vi "HandleTCPError.vi"(8 "error in (no error)":errorcluster, 10 "NoErrorMessage":refnum<class "Message.lvclass">, 11 "ServiceManager-Comms in":refnum<class "ServiceManager-Comms.lvclass">) -> (0 "error out":errorcluster, 3 "ServiceManager-Comms out":refnum<class "ServiceManager-Comms.lvclass">)   [LabVIEW 2020, in "ServiceManager-Comms.lvlib" / "ServiceManager-Comms.lvclass"]
uses:
  ServiceManager-Comms.lvclass
  C:/Program Files (x86)/National Instruments/LabVIEW 2020/vi.lib/ActorFramework/Actor/Actor.lvclass
  <vilib>/ActorFramework/Message/Message.lvclass
  ServiceManager-Comms Messages/WaitForConnect Msg/WaitForConnect Msg.lvclass
  C:/Program Files (x86)/National Instruments/LabVIEW 2020/vi.lib/ActorFramework/Message/Message.lvclass
  <vilib>/ActorFramework/Actor/Actor.lvclass/Actor.ctl
  <vilib>/ActorFramework/Message Enqueuer/Message Enqueuer.lvclass/Message Enqueuer.ctl
  <vilib>/ActorFramework/Message Enqueuer/Init from Existing Queue.vi
  <vilib>/ActorFramework/Message Enqueuer/Message Enqueuer.lvclass
  <vilib>/ActorFramework/Actor/Actor.lvclass
  C:/Users/taylo/Projects/g-go-service-fwrk/scratchpad/ServiceManagerBeta/ServiceManager/Nested/ServiceManager-Comms/ServiceManager-Comms Messages/WaitForConnect Msg/WaitForConnect Msg.lvclass
  C:/Users/taylo/Projects/g-go-service-fwrk/scratchpad/ServiceManagerBeta/ServiceManager/Nested/ServiceManager-Comms/ServiceManager-Comms.lvclass
  C:/Users/taylo/Projects/g-go-service-fwrk/scratchpad/ServiceManagerBeta/ServiceManager/Message Handling/Message Handling.lvclass
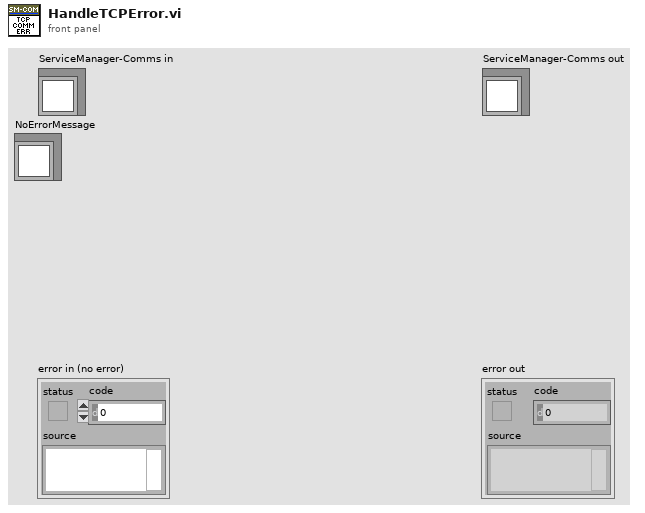
[diagram p1: front panel]
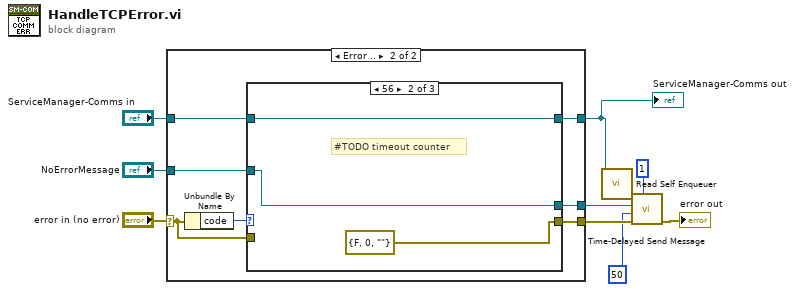
[diagram p0: block diagram]
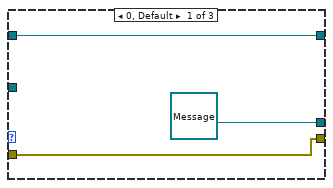
[diagram p3: hidden frame]
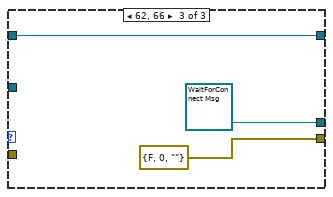
[diagram p4: hidden frame]
diagram:
  n1 = case shown="Error .." "error in (no error)" {
    selector: "error in (no error)" -> [w12 w15]
    tunnel: [w13 w18] -> w3
    tunnel: [w12 w17] -> w9
    tunnel: "ServiceManager-Comms in" -> [w13 w19]
    tunnel: [w11 w16] -> w7
    tunnel: "NoErrorMessage" -> [w11 w14]
    frame No Error {
    }
    frame Error {
      n2 = Unbundle By Name(w15) -> ("code"=w20:i32)
      n3 = case shown="56" w20 {
        tunnel: w19 -> [w23 w26 w29]
        tunnel: [w23 w26 w29] -> w18
        tunnel: [w21 errorcluster {"status"=FALSE, "code"=0, "source"=""} ("error IO") errorcluster {"status"=FALSE, "code"=0, "source"=""} ("error IO")] -> w17
        tunnel: [refnum<class "Message.lvclass"> refnum ("Message") w24 refnum<class "WaitForConnect Msg.lvclass"> refnum ("ServiceManager.lvlib:WaitForConnect Msg.lvclass")] -> w16
        tunnel: w15 -> [w21 _ _]
        tunnel: w14 -> [_ w24 _]
        frame 0, Default {
        }
        frame 56 {
          # "#TODO timeout counter"
        }
        frame 62, 66 {
        }
      }
    }
  }
  "ServiceManager-Comms out" <- w3
  n4 = call <vilib>:"Read Self Enqueuer.vi"("Actor"=w3) -> ("Self Enqueuer"=w10:refnum<class "Message Enqueuer.lvclass">)  [unwired: 10 in]
  n5 = call <vilib>:"Time-Delayed Send Message.vi"("# Copies (0 = infinite repeat)"=u32 1, "error in (no error)"=w9, "Milliseconds To Wait"=50, "Message"=w7, "Message Enqueuer"=w10) -> ("error out"=→"error out":errorcluster)  [unwired: 5 in, 1 out]
